vi "Check_FID_Response.vi"(3 "Mode":T5, 5 "Traverse line In":T2 {"Row Duration (mins)" format="%#.1f"; "Row No" min=0; "Trace Gas Concentration (%)" min=0.0 format="%#.2f"; "Emission Rate (l/min)" format="%#.2f"; "Tunnel Speed" format="%#.2f"; "Start X" format="%#.2f"; "Start Y" format="%#.2f"; "Start Z" format="%#.2f"; "End X" format="%#.2f"; "End Y" format="%#.2f"; "End Z" format="%#.2f"; "Averaging time (min)" min=0.0 format="%#.1f"}) -> (0 "Error Message":string, 1 "Status":T1, 2 "Traverse line Out":T2 {"Row Duration (mins)" format="%#.1f"; "Row No" min=0; "Trace Gas Concentration (%)" min=0.0 format="%#.2f"; "Emission Rate (l/min)" format="%#.2f"; "Tunnel Speed" format="%#.2f"; "Start X" format="%#.2f"; "Start Y" format="%#.2f"; "Start Z" format="%#.2f"; "End X" format="%#.2f"; "End Y" format="%#.2f"; "End Z" format="%#.2f"; "Averaging time (min)" min=0.0 format="%#.1f"})   [LabVIEW 2010]
uses:
  Controls/Setup.ctl
  Globals/Constants_global.vi
  Controls/Multi_run_mode.ctl
  Gen Trav/Multi_Run_Status.ctl
  Globals/Dynamic_call_global.ph.vi
  Globals/Meas_global.vi
  Controls/Post_Process.ctl
  Globals/Trav_pos_global.vi
  Controls/Save_Data.ctl
  ADAM Client/Sub VIs/ADAM Controls/Valco_valve_ph.ctl
  Gen Trav/Spacing.ctl
  Gen Trav/Traverse_cluster.ctl
  Controls/User_Specific_mode.ctl
panel:
  out "Speed Factor Array":dbl[](array[numeric]) format="%.2f"
  out "Raw Data Path":path
  # "X           Y            Z"
  # "Start"
  # "End"
  # "X           Y            Z"
  # "Start"
  # "End"
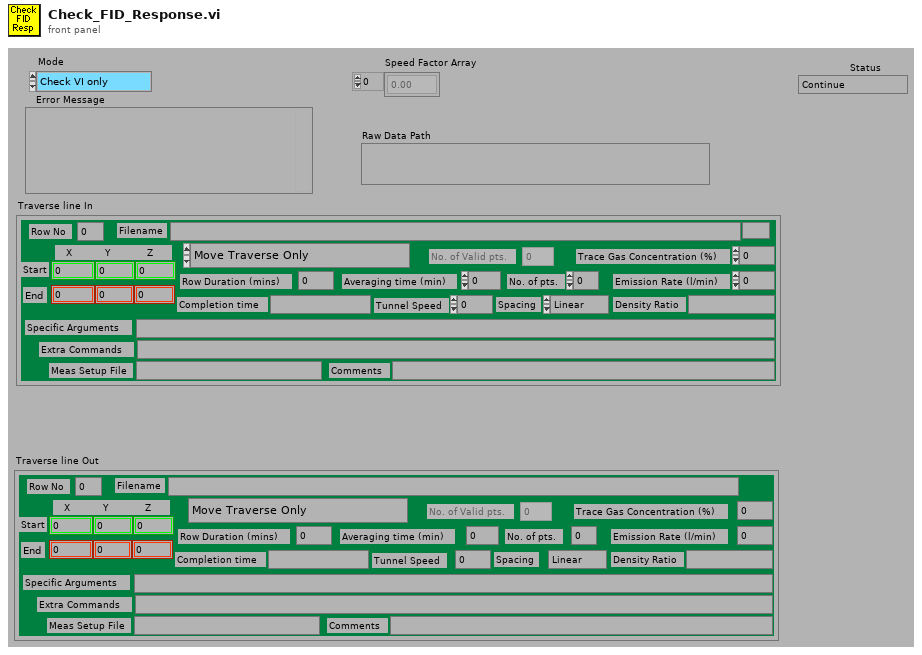
[diagram p1: front panel]
types:
  T1 = typedef "Multi_Run_Status.ctl" = enum16{"Continue", "Jump to Next Point", "Jump to Next Row", "Jump To Fall Back", "Terminate Run"}
  T2 = typedef "Traverse_cluster.ctl" = cluster{"Start X":dbl, "Start Y":dbl, "Start Z":dbl, "End X":dbl, "End Y":dbl, "End Z":dbl, "No. of pts.":i32, "Spacing":T3, "Filename":path, "Tunnel Speed":dbl, "Averaging time (min)":dbl, "Extra Commands":string, "Specific Arguments":string, "Emission Rate (l/min)":dbl, "Trace Gas Concentration (%)":dbl, "Density Ratio":string, "Comments":string, "Row No":i32, "Row Type Selector":T4, "Completion time":string, "Row Duration (mins)":dbl, "No. of Valid pts.":i32, "Meas Setup File":string}
  T3 = typedef "Spacing.ctl" = enum16{"Linear", "Log", "Gauss", "Specified", "N/A"}
  T4 = typedef "Multi_run_mode.ctl" = enum16{"Move Traverse Only", "Set Tunnel Speed Only", "Set Source Only", "Set Measurement Conditions", "Single Measurement", "Vertical Profile", "Lateral Profile", "Longitudinal Profile", "Explore Volume", "Multi-Axis Profile", "Auto Calibrate", "Meas Fast FID Bkgnd", "Check Beam Power", "Scanning Valve Measurement", "Run VI Named:", "Set ADAM Ch", "Wait (minutes)", "Send Message", "Synchronize With:", "Fall Back to this Row", "Turn Off Row Repeating", "Blank Row"}
  T5 = typedef "User_Specific_mode.ctl" = enum16{"Check VI only", "Run VI"}
  T6 = typedef "Setup.ctl" = enum16{"Run Program", "Show Setup", "Save Current Setup", "Setup Front Panel"}
  T7 = typedef "Save_Data.ctl" = enum16{"Save No Data", "Save Data"}
  T8 = typedef "Post_Process.ctl" = enum16{"Take New Data", "Post Process Raw Data File"}
  T9 = typedef "Status_Cluster.ctl" = cluster{"Status":T1, "Error Type":string, "Error Description":string}
  T10 = typedef "Valco_valve_ph.ctl" = u16
  T11 = typedef "Rendezvous RefNum" = refnum<k1>
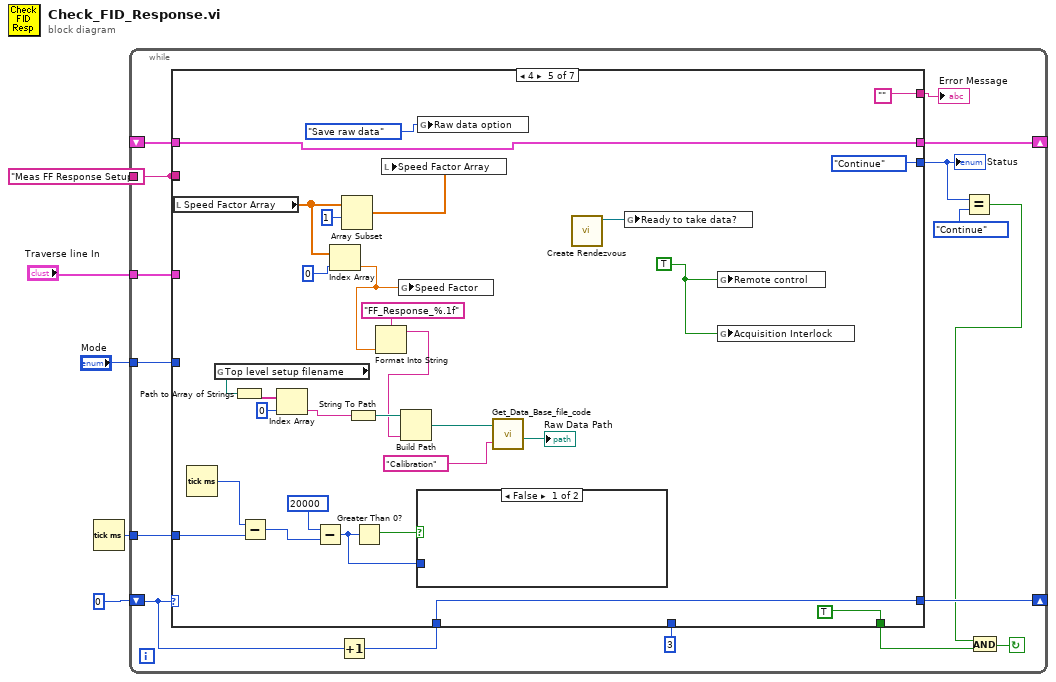
[diagram p0: block diagram]
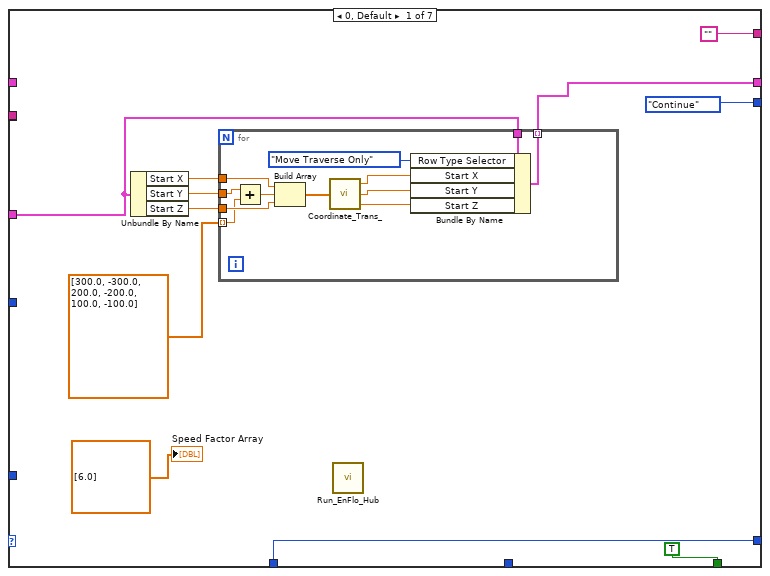
[diagram p2: hidden frame]
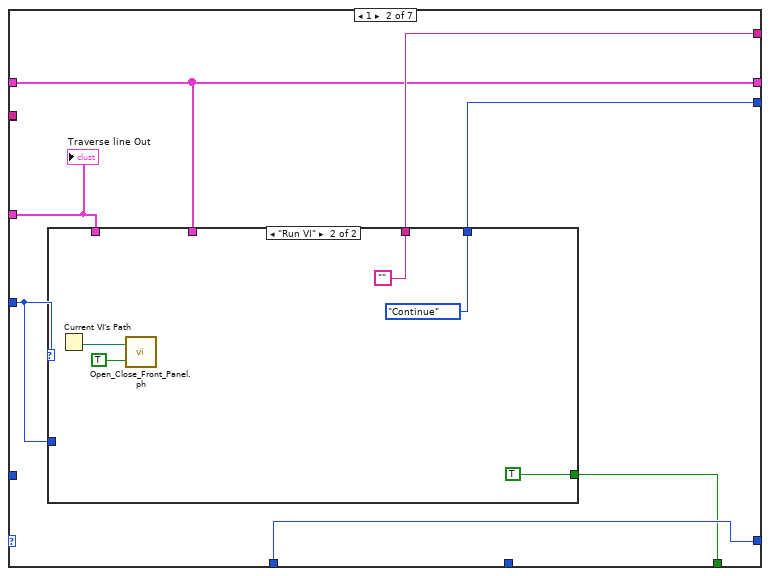
[diagram p3: hidden frame]
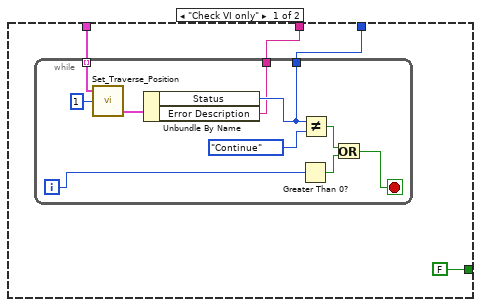
[diagram p4: hidden frame]
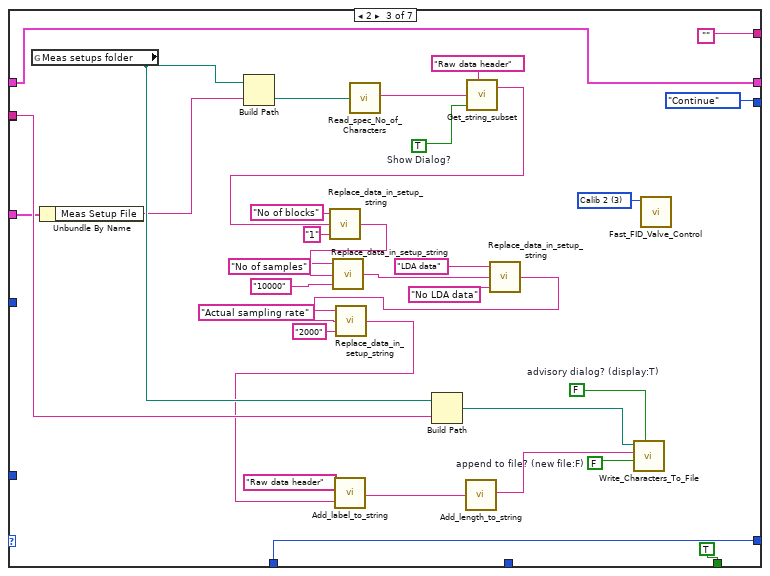
[diagram p5: hidden frame]
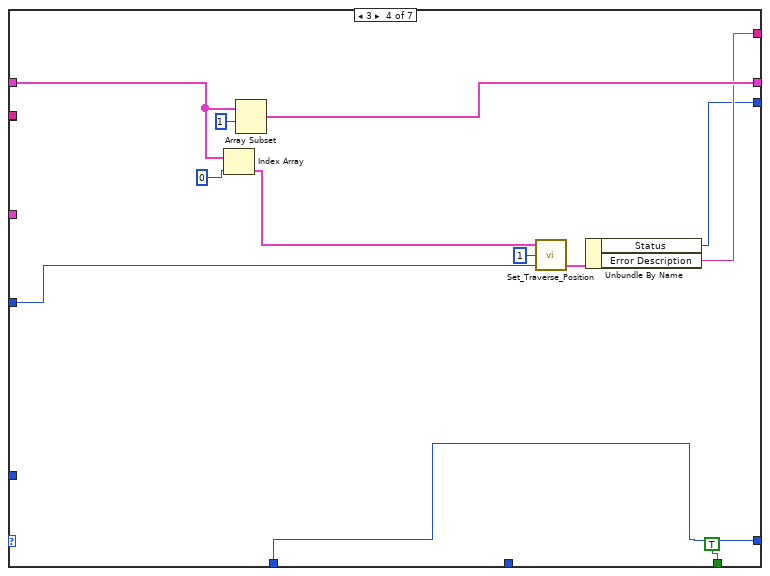
[diagram p6: hidden frame]
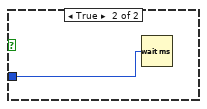
[diagram p7: hidden frame]
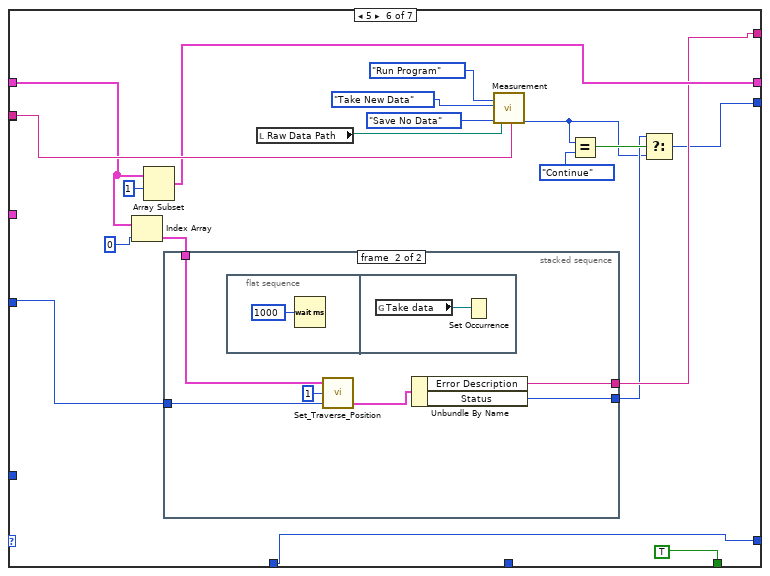
[diagram p8: hidden frame]
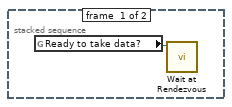
[diagram p9: hidden frame]
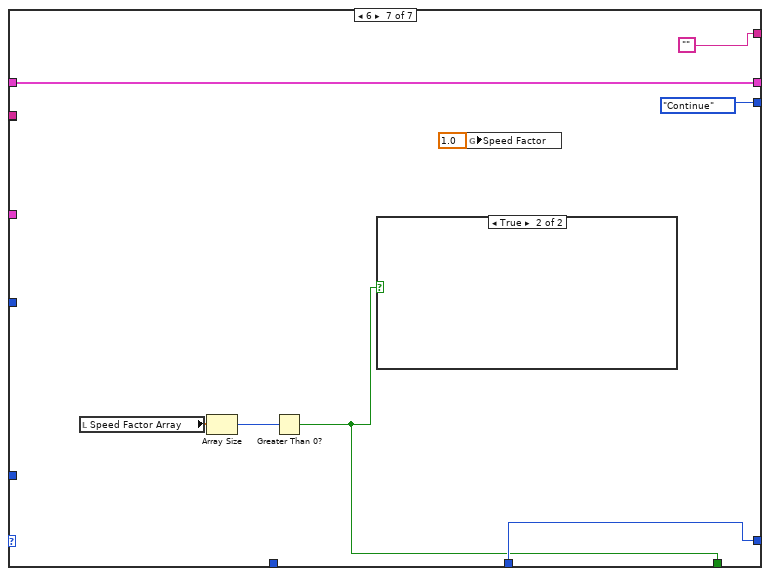
[diagram p10: hidden frame]
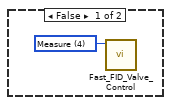
[diagram p11: hidden frame]
diagram:
  n1 = Tick Count (ms)() -> (millisecond timer value=w1:u32)
  n2 = while {
    tunnel: "Meas FF Response Setup" -> [w15]
    tunnel: "Traverse line In" -> [w19]
    tunnel: "Mode" -> [w20]
    shift-left: 0 -> [w21]
    shift-right: [w18] -> _
    shift-right: [w8] -> _
    shift-left: _ -> [w7]
    tunnel: w1 -> [w6]
    stop <- w9 continue-if-true
    n3 = Increment(x=w21) -> (x+1=w17:i32)
    n4 = case shown="4" w21 {
      tunnel: w19 -> [w23 w51 w76 _ _ _ _]
      tunnel: w20 -> [_ w50 _ w105 _ w161 _]
      tunnel: [TRUE ("Update Datum Powers?") w46 TRUE ("Update Datum Powers?") TRUE ("Update Datum Powers?") TRUE TRUE w174] -> w11
      tunnel: w17 -> [w32 w47 w103 w104 w141 w163 _]
      tunnel: [w32 w47 w103 w104 w141 w163 w175] -> w18
      tunnel: w15 -> [_ _ w90 _ _ _ _]
      tunnel: ["" w48 "" w107 "" w155 ""] -> w16
      tunnel: w15 -> [_ _ _ _ _ w162 _]
      tunnel: 3 ("t") -> [_ _ _ _ _ _ w175]
      tunnel: [Multi_Run_Status."Continue" ("Status") w49 Multi_Run_Status."Continue" ("Status") w106 Multi_Run_Status."Continue" ("Status") w150 Multi_Run_Status."Continue" ("Status")] -> w12
      tunnel: [w22 w45 w72 w111 w123 w156 w178] -> w8
      tunnel: w7 -> [_ w45 w72 w112 w123 w158 w178]
      tunnel: w6 -> [_ _ _ _ w120 _ _]
      frame 0, Default {
        n5 = Unbundle By Name(w23) -> ("Start X"=w26:dbl, "Start Y"=w27:dbl, "Start Z"=w25:dbl)
        n6 = for {
          tunnel: w23 -> [w42]
          tunnel: w27 -> [w40]
          tunnel: w26 -> [w39]
          tunnel: w25 -> [w38]
          tunnel: dbl[] [300.0, -300.0, 200.0, -200.0, 100.0, -100.0] ("Speed Factor Array") -> [w34] mode=indexing
          tunnel: [w33] -> w22 mode=indexing
          n7 = Add(x=w40, y=w34) -> (x+y=w41:dbl)
          n8 = Build Array(w39, w41, w38) -> (w43:dbl[])
          n9 = call "Coordinate_Trans_.vi"("Input Position"=w43) -> ("X"=w37:dbl, "Y"=w36:dbl, "Z"=w35:dbl)
          n10 = Bundle By Name(cluster=w42, "Row Type Selector"=Multi_run_mode."Move Traverse Only", "Start X"=w37, "Start Y"=w36, "Start Z"=w35) -> (w33:T2)
        }
        n11 = call "Run_EnFlo_Hub.vi"() -> ()  [unwired: 8 out]
        "Speed Factor Array" <- dbl[] [6.0] ("Speed Factor Array")
      }
      frame 1 {
        n12 = case shown="\"Run VI\"" w50 {
          tunnel: w51 -> [_ _]
          tunnel: w50 -> [_ _]
          tunnel: [w55 Multi_Run_Status."Continue" ("Status")] -> w49
          tunnel: [w54 ""] -> w48
          tunnel: [FALSE ("Update Datum Powers?") TRUE ("Update Datum Powers?")] -> w46
          tunnel: w45 -> [w52 _]
          frame "Check VI only" {
            n13 = while {
              tunnel: [w58] -> w55
              tunnel: [w57] -> w54
              tunnel: w52 -> [w56] mode=indexing
              i -> [w59]
              stop <- w60 stop-if-true
              n14 = call "Set_Traverse_Position.vi"("Currently on Point"=1, "Traverse line"=w56) -> ("Status Cluster"=w64:T9)  [unwired: 1 in, 2 out]
              n15 = Unbundle By Name(w64) -> ("Status"=w58:T1, "Error Description"=w57:string)
              n16 = Greater Than 0?(x=w59) -> (x > 0?=w62:bool)
              n17 = Not Equal?(x=w58, y=Multi_Run_Status."Continue" ("Status")) -> (x != y?=w61:bool)
              n18 = Or(x=w61, y=w62) -> (x .or. y?=w60:bool)
            }
          }
          frame "Run VI" {
            n19 = Current VI's Path() -> (path=w69:path)
            n20 = call "Open_Close_Front_Panel.ph.vi"("Front Panel Window:Open"=TRUE, "VI path"=w69) -> ()  [unwired: 2 out]
          }
        }
        "Traverse line Out" <- w51
      }
      frame 2 {
        w71 = T10 3 items=["", "Zero Air", "Calib 1", "Calib 2", "Measure"] ("Requested Position")
        w96 = FALSE  # advisory dialog? (display:T)
        w97 = FALSE  # append to file? (new file:F)
        w98 = TRUE  # Show Dialog?
        n21 = global read "Constants_global.vi" "Meas setups folder"() -> (w91:path)
        n22 = Unbundle By Name(w76) -> ("Meas Setup File"=w75:string)
        n23 = Build Path(base path=w91, name or relative path=w75) -> (appended path=w99:path)
        n24 = call "Read_spec_No_of_Characters.vi"("Filename"=w99) -> ("character string"=w100:string)  [unwired: 1 out]
        n25 = Build Path(base path=w91, name or relative path=w90) -> (appended path=w92:path)
        n26 = call "Get_string_subset.vi"("Show Dialog?"=w98, "String to split"=w100, "File Label"="Raw data header") -> ("Output string"=w88:string)  [unwired: 1 out]
        n27 = call "Replace_data_in_setup_string.vi"("New data string"="1", "Input string"=w88, "Variable name"="No of blocks") -> ("Appended string"=w86:string)
        n28 = call "Replace_data_in_setup_string.vi"("New data string"="10000", "Input string"=w86, "Variable name"="No of samples") -> ("Appended string"=w78:string)
        n29 = call "Replace_data_in_setup_string.vi"("New data string"="No LDA data", "Input string"=w78, "Variable name"="LDA data" ("Label for characters")) -> ("Appended string"=w77:string)
        n30 = call "Replace_data_in_setup_string.vi"("New data string"="2000", "Input string"=w77, "Variable name"="Actual sampling rate") -> ("Appended string"=w85:string)
        n31 = call "Add_label_to_string.vi"("String to write"=w85, "File Label"="Raw data header") -> ("Output string"=w93:string)
        n32 = call "Add_length_to_string.vi"("String in"=w93) -> ("String out"=w95:string)
        n33 = call "Write_Characters_To_File.vi"("file path (dialog if empty)"=w92, "advisory dialog? (display:T)"=w96, "character string"=w95, "append to file? (new file:F)"=w97) -> ()  [unwired: 1 in, 4 out]
        n34 = call "Fast_FID_Valve_Control.vi"("Requested Position"=w71) -> ()  [unwired: 7 out]
      }
      frame 3 {
        n35 = Index Array(array=w112, index=0 ("Index")) -> (element=w110:T2)
        n36 = Array Subset(array=w112, index=1 ("Array Index")) -> (w111:T2[])  [unwired: 1 in]
        n37 = call "Set_Traverse_Position.vi"("Simulate/Run"=w105, "Currently on Point"=1, "Traverse line"=w110) -> ("Status Cluster"=w115:T9)  [unwired: 2 out]
        n38 = Unbundle By Name(w115) -> ("Status"=w106:T1, "Error Description"=w107:string)
      }
      frame 4 {
        w142 = TRUE ("Remote control")
        n39 = local read "Speed Factor Array"() -> (w131:dbl[])
        n40 = Tick Count (ms)() -> (millisecond timer value=w121:u32)
        n41 = global read "Trav_pos_global.vi" "Top level setup filename"() -> (w140:path)
        n42 = Path to Array of Strings(0:w140) -> (2:w139:string[])  [unwired: 1 out]
        n43 = Subtract(x=w121, y=w120) -> (x-y=w118:u32)
        n44 = Index Array(array=w139, index=0 ("Index")) -> (element=w135:string)
        n45 = Subtract(x=20000, y=w118) -> (x-y=w116:u32)
        n46 = Index Array(array=w131, index=0 ("Index")) -> (element=w129:dbl)
        n47 = Array Subset(array=w131, index=1 ("Array Index")) -> (w130:dbl[])  [unwired: 1 in]
        n48 = String To Path(string=w135) -> (path=w137:path)
        n49 = Greater Than 0?(x=w116) -> (x > 0?=w117:bool)
        n50 = Format Into String(format string="FF_Response_%.1f" ("Format String"), w129) -> (resulting string=w127:string)  [unwired: 2 in, 1 out]
        n51 = local write "Speed Factor Array"(w130) -> ()
        n52 = global write "Trav_pos_global.vi" "Speed Factor"(w129) -> ()
        n53 = Build Path(base path=w137, name or relative path=w127) -> (appended path=w136:path)
        n54 = case shown="False" w117 {
          tunnel: w116 -> [_ w145]
          frame False {
          }
          frame True {
            n55 = Wait (ms)(milliseconds to wait=w145) -> ()  [unwired: 1 out]
          }
        }
        n56 = global write "Meas_global.vi" "Raw data option"(enum16{"Save raw data", "Raw data not saved"}."Save raw data" ("Raw data option")) -> ()
        n57 = call "Get_Data_Base_file_code.vi"("Results Filename"=w136, "Data Type"="Calibration") -> ("Raw Data File Name"=→"Raw Data Path":path)  [unwired: 3 out]
        n58 = call <vilib>:"Create Rendezvous.vi"() -> ("rendezvous"=w143:T11)  [unwired: 2 in, 5 out]
        n59 = global write "Dynamic_call_global.ph.vi" "Ready to take data?"(w143) -> ()
        n60 = global write "Meas_global.vi" "Remote control"(w142) -> ()
        n61 = global write "Dynamic_call_global.ph.vi" "Acquisition Interlock"(w142) -> ()
      }
      frame 5 {
        n62 = Index Array(array=w158, index=0 ("Index")) -> (element=w157:T2)
        n63 = Array Subset(array=w158, index=1 ("Array Index")) -> (w156:T2[])  [unwired: 1 in]
        n64 = stacked-sequence {
          tunnel: w161 -> [_ w170]
          tunnel: w157 -> [_ w169]
          tunnel: [_ w167] -> w155
          tunnel: [_ w166] -> w152
          frame #0 {
            n65 = global read "Dynamic_call_global.ph.vi" "Ready to take data?"() -> (w165:T11)
            n66 = call <vilib>:"Wait at Rendezvous.vi"("rendezvous"=w165) -> ()  [unwired: 2 in, 5 out]
          }
          frame #1 {
            n67 = flat-sequence {
              frame #0 {
                n68 = Wait (ms)(milliseconds to wait=u32 1000) -> ()  [unwired: 1 out]
              }
              frame #1 {
                n69 = global read "Dynamic_call_global.ph.vi" "Take data"() -> (w173:refnum<k4>)
                n70 = Set Occurrence(w173) -> ()
              }
            }
            n71 = call "Set_Traverse_Position.vi"("Simulate/Run"=w170, "Currently on Point"=1, "Traverse line"=w169) -> ("Status Cluster"=w168:T9)  [unwired: 2 out]
            n72 = Unbundle By Name(w168) -> ("Error Description"=w167:string, "Status"=w166:T1)
          }
        }
        n73 = local read "Raw Data Path"() -> (w148:path)
        n74 = call "Measurement.vi"("setup"=Setup."Run Program", "Post Process"=Post_Process."Take New Data", "File"=Save_Data."Save No Data", "Raw data file"=w148, "Setup filename"=w162) -> ("Status Out"=w151:T1)  [unwired: 2 in, 12 out]
        n75 = Equal?(x=w151, y=Multi_Run_Status."Continue" ("Status")) -> (x = y?=w153:bool)
        n76 = Select(t=w152, s=w153, f=w151) -> (s? t:f=w150:T1)
      }
      frame 6 {
        n77 = local read "Speed Factor Array"() -> (w181:dbl[])
        n78 = Array Size(array=w181) -> (size(s)=w180:i32)
        n79 = Greater Than 0?(x=w180) -> (x > 0?=w174:bool)
        n80 = case shown="True" w174 {
          frame False {
            w182 = T10 4 items=["", "Zero Air", "Calib 1", "Calib 2", "Measure"] ("Requested Position")
            n81 = call "Fast_FID_Valve_Control.vi"("Requested Position"=w182) -> ()  [unwired: 7 out]
          }
          frame True {
          }
        }
        n82 = global write "Trav_pos_global.vi" "Speed Factor"(1.0 ("Speed Factor")) -> ()
      }
    }
    "Error Message" <- w16
    "Status" <- w12
    n83 = Equal?(x=w12, y=Multi_Run_Status."Continue" ("Status")) -> (x = y?=w10:bool)
    n84 = And(x=w10, y=w11) -> (x .and. y?=w9:bool)
  }
